vi "send single action command.vi"(8 "error in":errorcluster, 9 "engine name":string, 10 "command":T1, 11 "message queue in":T2) -> (0 "error out":errorcluster, 3 "message queue out":T2)   [LabVIEW 2013, in "module execution process.lvlib"]
uses:
  module execution process.lvlib
  <vilib>/NI/AMC/Message Queue.ctl
  <vilib>/NI/AMC/Message.ctl
  <vilib>/NI/Tools/Keyed Array/KeyedArray.ctl
  command commands to rtexe process.ctl
  <vilib>/NI/AMC/Create Single Message.vi
  <vilib>/NI/AMC/Update Message Routing Info.vi
  <vilib>/NI/AMC/Send Message.vi
  <vilib>/NI/AMC/AMC.lvlib
  <vilib>/NI/Tools/Keyed Array/Tools_KeyedArray.lvlib
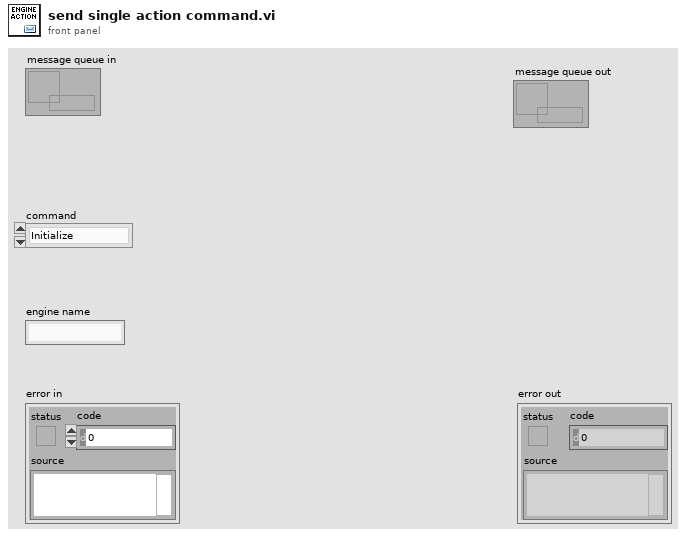
[diagram p1: front panel]
types:
  T1 = typedef "module execution process.lvlib/command commands to rtexe process.ctl" = enum16{"Initialize", "Load from File", "Load from String", "Open All Engines", "Open Single Engine", "Initialize All Engines", "Initialize Single Engine", "Start All", "Start Single", "Pause All", "Pause Single", "Stop All", "Stop Single", "Close All", "Close Single", "Set Safe State All", "Set Safe State Single", "Get Status", "Exit", "Error", "Load Bitfile", "Unload Bitfile", "Add Search Paths"}
  T2 = typedef "AMC.lvlib/Message Queue.ctl" = refnum<queue>
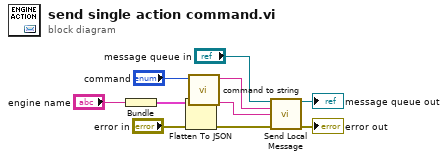
[diagram p0: block diagram]
diagram:
  n1 = Bundle("engine name"="engine name") -> (w1:cluster{"engine name":string})  [unwired: 1 in]
  n2 = Flatten To JSON(anything=w1, error in (no error)="error in") -> (JSON string=w3:string, 11:w4:errorcluster)  [unwired: 1 in]
  n3 = call "command to string.vi"("commands"="command") -> ("command string"=w6:string)  [unwired: 10 in]
  n4 = call <vilib>:"Send Local Message.vi"("message queue in"="message queue in", "message name"=w6, "message value"=w3, "error in"=w4) -> ("message queue out"=→"message queue out":T2, "error out"=→"error out":errorcluster)  [unwired: 9 in, 1 out]
